vi "TSM Relay Control Per-Site.vi"(0 "Relay TSM In":T1, 2 "Settling Time (s)":dbl, 5 "Per-Site Relay Actions":T3[](array[typedef]) items=["Open Relay"=20, "Close Relay"=21], 11 "error in":errorcluster) -> (15 "error out":errorcluster)   [LabVIEW 2020]
doc: "Performs the specified per-site relay actions on all specified relays. \n\n-If the action array has one element the function maps it to all sites\n-If the array is an even multiple size of the number of sites it maps the array multiple times (used to expand across sites)\n-If the action array is not an even multiple size the function maps the array and emits a warning\n-If the action array is larger than the sites it gets shortened and the function emits a warning"
uses:
  <vilib>/NI_TestStand_SemiconductorModule/NI_TestStand_Semiconductor_Module.lvlibp/1abvi3w/instr.lib/niSwitch/niswitch.llb/niSwitch Relay Action.ctl
  Pin Map/TSM Relay.ctl
  <vilib>/NI_TestStand_SemiconductorModule/NI_TestStand_Semiconductor_Module.lvlibp/PinMap/General/SemiconductorModuleContext.ctl
  ee22f031-ec38-4f28-81b6-ff4c7fb4bdad.vi
  <vilib>/Utility/error.llb/Error Cluster From Error Code.vi
  <vilib>/NI_TestStand_SemiconductorModule/NI_TestStand_Semiconductor_Module.lvlibp/PinMap/Relay Driver/ControlRelaysSingleAction.vi
  <vilib>/NI_TestStand_SemiconductorModule/NI_TestStand_Semiconductor_Module.lvlibp
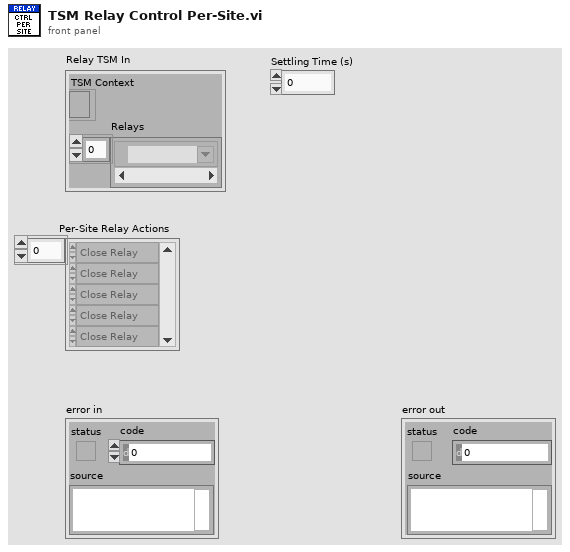
[diagram p1: front panel]
types:
  T1 = typedef "TSM Relay.ctl" = cluster{"TSM Context":T2, "Relays":tag[]}
  T2 = typedef "NI_TestStand_Semiconductor_Module.lvlibp/SemiconductorModuleContext.ctl" = refnum<k7>
  T3 = typedef "NI_TestStand_Semiconductor_Module.lvlibp/niSwitch Relay Action.ctl" = i32
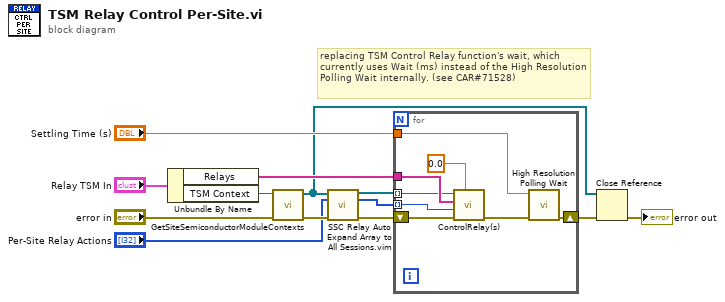
[diagram p0: block diagram]
diagram:
  # "replacing TSM Control Relay function's wait, which currently uses Wait (ms) instead of the High Resolution Polling Wait internally. (see CAR#71528)"
  n1 = Unbundle By Name("Relay TSM In") -> ("Relays"=w9:tag[], "TSM Context"=w10:T2)
  n2 = call <vilib>:"GetSiteSemiconductorModuleContexts.vi"("error in (no error)"="error in", "Semiconductor Module Context"=w10) -> ("error out"=w8:errorcluster, "Site Semiconductor Module Contexts"=w1:T2[])  [unwired: 8 in]
  n3 = call "SSC Relay Auto Expand Array to All Sessions.vim"("Relay TSM In"=w1, "Data In"="Per-Site Relay Actions", "error in"=w8) -> ("Relay TSM Out"=w2:T2[], "Data Out"=w6:T3[], "error out"=w4:errorcluster)  [unwired: 10 in]
  n4 = for {
    tunnel: "Settling Time (s)" -> [w16]
    tunnel: w6 -> [w14] mode=indexing
    tunnel: w9 -> [w20]
    shift-right: [w17] -> w5
    shift-left: w4 -> [w21]
    tunnel: w2 -> [w18] mode=indexing
    n5 = call-poly <vilib>:"ControlRelay(s).vi"("Wait (s)"=0.0, "error in (no error)"=w21, "Relay Action"=w14, "Relays"=w20, "Semiconductor Module Context"=w18) -> ("error out"=w19:errorcluster)  [unwired: 5 in, 1 out]
    n6 = call <vilib>:"High Resolution Polling Wait.vi"("error in (no error)"=w19, "seconds to wait"=w16) -> ("error out"=w17:errorcluster)  [unwired: 9 in]
  }
  n7 = Close Reference(reference=w1, error in (no error)=w5) -> (error out=→"error out":errorcluster)
